vi "Flush.vi"(11 "POTTypedCircularBuffer in":refnum<class "ErrorLogBuffer.lvclass">) -> (3 "POTTypedCircularBuffer out":refnum<class "ErrorLogBuffer.lvclass">)   [LabVIEW 2024, in "ErrorLogBuffer.lvclass"]
uses:
  ErrorLogBuffer.lvclass
  ErrorLogBuffer.lvclass/ErrorLogBuffer.ctl
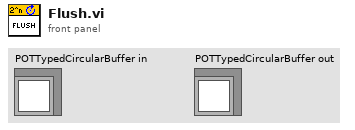
[diagram p1: front panel]
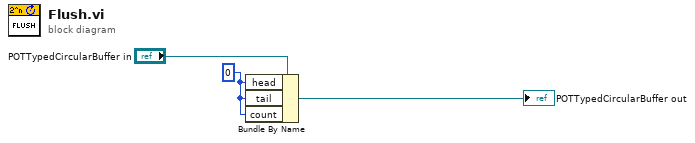
[diagram p0: block diagram]
diagram:
  w1 = 0 ("head")
  n1 = Bundle By Name(cluster="POTTypedCircularBuffer in", "head"=w1, "tail"=w1, "count"=w1) -> (→"POTTypedCircularBuffer out":refnum<class "ErrorLogBuffer.lvclass">)
